vi "Get.vi"(11 "Entity in":refnum<class "Entity.lvclass">) -> (2 "Value":refnum<class "Entity.lvclass">)   [LabVIEW 2022 SP3, in "Conditum.lvlib" / "Columns.lvlib" / "Entity.lvclass"]
uses:
  Entity.lvclass
  Entity.lvclass/Entity.ctl
  Entity/Entity.lvclass
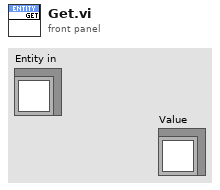
[diagram p1: front panel]
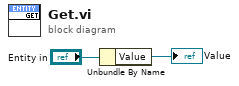
[diagram p0: block diagram]
diagram:
  n1 = Unbundle By Name("Entity in") -> ("Value"=→"Value":refnum<class "Entity.lvclass">)
